vi "Convert DOF To Maximum.vi"(10 "Data Output Format":T1=enum."8-bit Mode" caption="NewVal") -> (2 "Data Maximum":dbl)   [LabVIEW 2026, in "MicroPulse_Driver.lvlib"]
uses:
  MicroPulse_Driver.lvlib
  Datatypes/MP - data output format.ctl
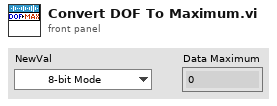
[diagram p1: front panel]
types:
  T1 = typedef "MicroPulse_Driver.lvlib/MP - data output format.ctl" = enum16{"", "8-bit Mode", "10-bit Mode", "12-bit Mode", "16-bit Mode", "8-bit Log Mode", "12-bit Packed Mode"}
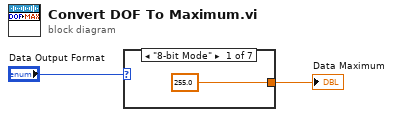
[diagram p0: block diagram]
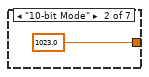
[diagram p2: hidden frame]
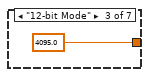
[diagram p3: hidden frame]
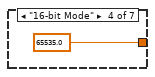
[diagram p4: hidden frame]
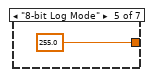
[diagram p5: hidden frame]
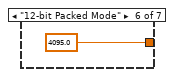
[diagram p6: hidden frame]
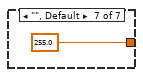
[diagram p7: hidden frame]
diagram:
  n1 = case shown="\"8-bit Mode\"" "Data Output Format" {
    tunnel: [255.0 ("Y Scale.Range:Maximum") 1023.0 ("Y Scale.Range:Maximum") 4095.0 ("Y Scale.Range:Maximum") 65535.0 ("Y Scale.Range:Maximum") 255.0 ("Y Scale.Range:Maximum") 4095.0 ("Y Scale.Range:Maximum") 255.0 ("Y Scale.Range:Maximum")] -> w1
    frame "8-bit Mode" {
    }
    frame "10-bit Mode" {
    }
    frame "12-bit Mode" {
    }
    frame "16-bit Mode" {
    }
    frame "8-bit Log Mode" {
    }
    frame "12-bit Packed Mode" {
    }
    frame "", Default {
    }
  }
  "Data Maximum" <- w1
